vi "Initialise Connection--SubVI.vi"(7 "Client ID":string="BTSMQTTBRIDGE", 8 "error in (no error)":errorcluster, 10 "remote port (1883)":u16=80, 11 "address (localhost)":string="localhost") -> (0 "error out":errorcluster, 3 "MQTT_Base out":refnum<class "Client.lvclass">)   [LabVIEW 2024, in "MQTTClient.lvlib"]
doc: "<b>Note:</b> This VI was modified by the <b>Validate DQMH Module</b> tool to turn off automatic error handling."
uses:
  MQTTClient.lvlib
  <vilib>/LabVIEW Open Source Project/MQTT Client/Client class/Client.lvclass
  C:/Program Files/National Instruments/LabVIEW 2025/vi.lib/LabVIEW Open Source Project/MQTT Connection/MQTT_Base/Base Class/MQTT_Base.lvclass
  <vilib>/LabVIEW Open Source Project/MQTT Connection/MQTT_Base/Base Class/MQTT_Base.lvclass
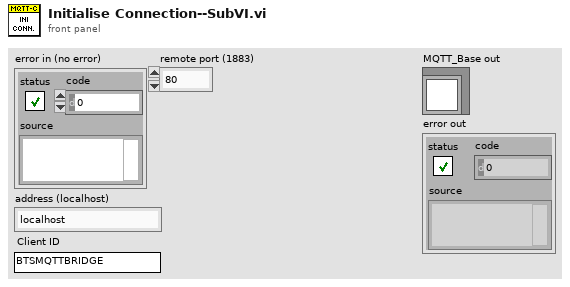
[diagram p1: front panel]
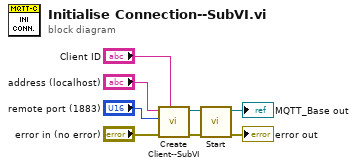
[diagram p0: block diagram]
diagram:
  n1 = call "Create Client--SubVI.vi"("Client ID"="Client ID", "error in (no error)"="error in (no error)", "remote port (1883)"="remote port (1883)", "address (localhost)"="address (localhost)") -> ("error out"=w5:errorcluster, "MQTT_Base out"=w4:refnum<class "Client.lvclass">)  [unwired: 6 in]
  n2 = call <vilib>:"Start.vi"("error in (no error)"=w5, "MQTT_Base in"=w4) -> ("error out"=→"error out":errorcluster, "MQTT_Base out"=→"MQTT_Base out":refnum<class "Client.lvclass">)  [unwired: 7 in, 1 out]
